vi "打印前面板R567B.vi"(10 "字符串":string, 11 "二维码图片":picture) -> ()   [LabVIEW 2020]
panel:
  out "字符串2":string
  out "二维码图片2":picture
  # "201000437AA"
  # "S"
  # "3404ABE"
  # "4BS"
  # "SW VER:00.02.00"
  # "HW VER:0.0.1"
  # "CHN"
  # "SE CONF:07"
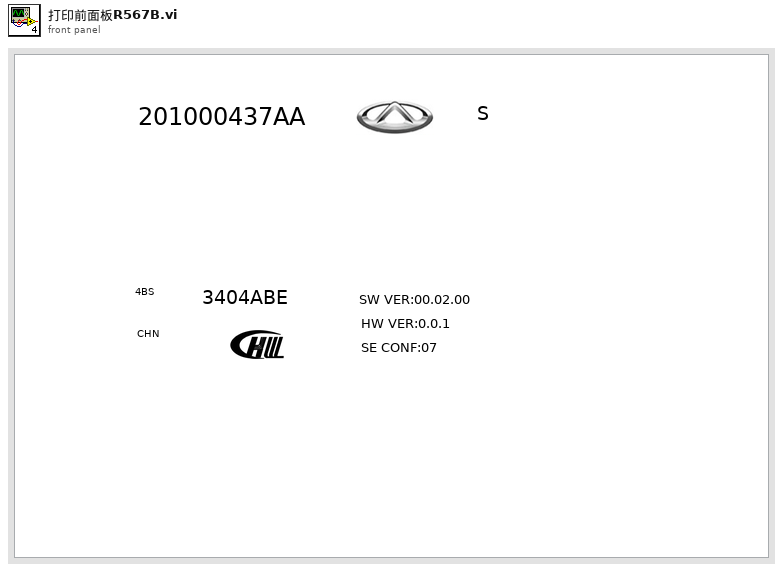
[diagram p1: front panel]
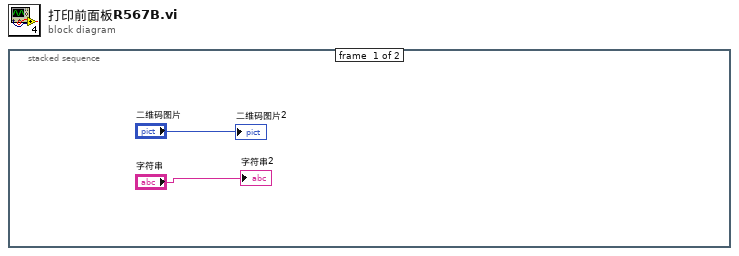
[diagram p0: block diagram]
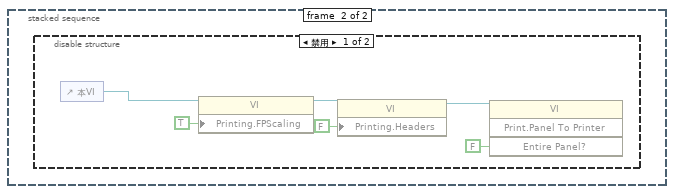
[diagram p2: hidden frame]
diagram:
  n1 = stacked-sequence {
    frame #0 {
      "二维码图片2" <- "二维码图片"
      "字符串2" <- "字符串"
    }
    frame #1 {
      n2 = disable-structure shown="禁用" {
        frame Disabled {
          n3 = control-ref of="本VI"() -> (w8:refnum<vi>)
          n4 = property class="VI"(reference=w8, "Printing.FPScaling"=TRUE ("打印:前面板缩放？")) -> (reference out=w6:refnum<vi>)  [unwired: 1 in, 1 out]
          n5 = property class="VI"(reference=w6, "Printing.Headers"=FALSE ("打印:页眉？")) -> (reference out=w4:refnum<vi>)  [unwired: 1 in, 1 out]
          n6 = invoke class="VI" method="Print.Panel To Printer"(reference=w4, "Entire Panel?"=FALSE ("整个前面板？")) -> ()  [unwired: 2 in, 4 out]
        }
        frame Enabled {
        }
      }
    }
  }
